vi "Begin.vi"(8 "error in":errorcluster) -> (0 "error out":errorcluster)   [LabVIEW 2016]
doc: "Called before other user functions, this VI is expected to open initial I/O refnums, load in file data, and do all program initialization. Notice that the <B>error out</B> terminal is simply used for data flow. Wiring it to other structures or subVIs ensures that this VI runs first."
uses:
  <vilib>/Rock Robotics/WPI/DriverStation/WPI_DriverStationRobotMode2.ctl
  <vilib>/Rock Robotics/WPI/Joystick/WPI_JoystickDeviceEnum.ctl
  <vilib>/Rock Robotics/SystemInterfaces/DIO/FPGA_DIOPWMChannel.ctl
  <vilib>/Rock Robotics/WPI/SafetyOutput/WPI_SafetyOutputConfigMenu.ctl
  <vilib>/Rock Robotics/WPI/ThirdParty/CanMotor/TalonSRX/WPI_CANTalonSRX_APIControlMode.ctl
  <vilib>/Rock Robotics/WPI/ThirdParty/CanMotor/TalonSRX/WPI_CANTalonSRX_APIFeedbackSelect.ctl
  Robot Global Data.vi
  <vilib>/Rock Robotics/Network Tables/NT Write String Array.vi
  <vilib>/Rock Robotics/Network Tables/NT Write String.vi
  5492_DriveOrientation.vi
  5492_OrientationButtonPress.vi
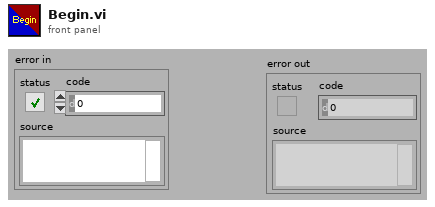
[diagram p1: front panel]
types:
  T1 = typedef "FPGA_DIOPWMChannel.ctl" = enum8{"PWM 0", "PWM 1", "PWM 2", "PWM 3", "PWM 4", "PWM 5", "PWM 6", "PWM 7", "PWM 8", "PWM 9", "PWM MXP 0", "PWM MXP 1", "PWM MXP 2", "PWM MXP 3", "PWM MXP 4", "PWM MXP 5", "PWM MXP 6", "PWM MXP 7", "PWM MXP 8", "PWM MXP 9", "Invalid"}
  T2 = typedef "WPI_CANTalonSRX_APIControlMode.ctl" = enum8{"Percent VBus", "Speed", "Position", "Slave", "Unchanged / Invalid", "Voltage Compensation", "Current", "Motion Profile", "Motion Magic"}
  T3 = typedef "WPI_CANTalonSRX_APIFeedbackSelect.ctl" = enum16{"Digital Quadrature Encoder", "Analog Potentiometer", "Analog Encoder", "Count on Quad-A (Rising-Edge)", "Count on Quad-A (Falling-Edge)", "CTR Magnetic Enc (Absolute)", "CTR Magnetic Enc (Relative)", "Pulse Width"}
  T4 = typedef "WPI_JoystickDeviceEnum.ctl" = enum16{"USB 0", "USB 1", "USB 2", "USB 3", "USB 4", "USB 5"}
  T5 = typedef "WPI_SafetyOutputConfigMenu.ctl" = enum16{"Enable", "Disable"}
  T6 = typedef "WPI_DriverStationRobotMode2.ctl" = enum16{"Autonomous Disabled", "Autonomous Enabled", "Teleop Disabled", "Teleop Enabled", "Disconnected", "Finish", "Test Disabled", "Test Enabled", "Emergency Stopped"}
  T7 = typedef "WPI_JoystickDevRef.ctl" = cluster{"Device":T4}
  T8 = typedef "WPI_MotorControlDeviceRef.ctl" = cluster{"DeviceStatus":errorcluster, "Type":T9, "PWM":cluster{"PWM Channel":T1, "DeadBand":T10}, "CAN":cluster{"Device Number":u8, "SetOutput VI Ref":variant, "GetOutput VI Ref":variant, "Enable VI Ref":variant, "Disable VI Ref":variant, "Data":variant}, "Invert":bool}
  T9 = typedef "WPI_MotorControlType.ctl" = enum16{"PWM", "CAN"}
  T10 = typedef "WPI_PWMDeadband.ctl" = cluster{"Name":string, "maxPositivePwm":i32, "minPositivePwm":i32, "centerPwm":i32, "maxNegativePwm":i32, "minNegativePwm":i32, "angularRange":u16}
  T11 = typedef "WPI_RobotDriveDevRef.ctl" = cluster{"DevStatus":errorcluster, "Motors[]":T8[], "Square Inputs":bool, "Max Output":dbl}
  T12 = typedef "WPI_PWMDeviceRef.ctl" = cluster{"DeviceStatus":errorcluster, "PWM Channel":T1}
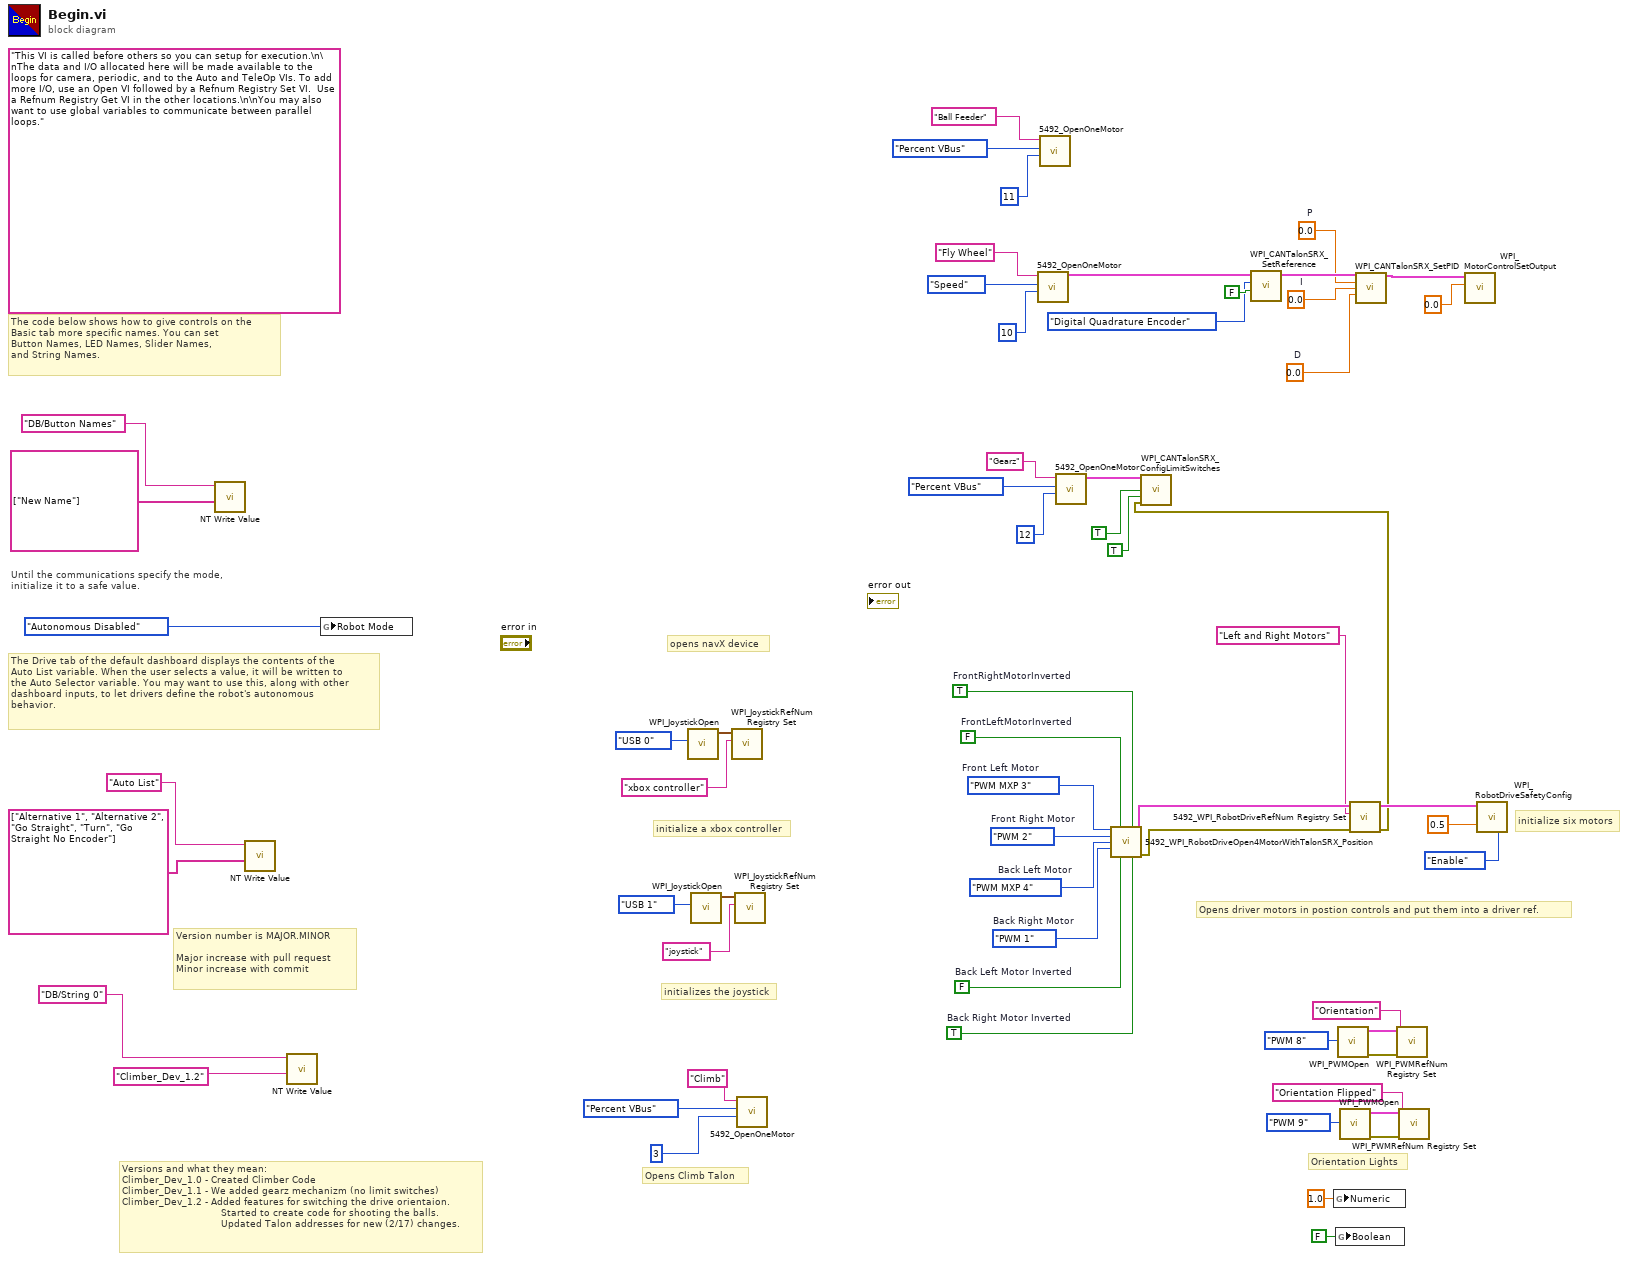
[diagram p0: block diagram]
diagram:
  w16 = 0.0  # D
  w17 = 0.0  # I
  w18 = 0.0  # P
  w43 = TRUE  # Back Right Motor Inverted
  w44 = FALSE  # Back Left Motor Inverted
  w45 = FPGA_DIOPWMChannel."PWM MXP 4"  # Back Left Motor
  w51 = FPGA_DIOPWMChannel."PWM 1"  # Back Right Motor
  w52 = FPGA_DIOPWMChannel."PWM 2"  # Front Right Motor
  w53 = FPGA_DIOPWMChannel."PWM MXP 3"  # Front Left Motor
  w50 = FALSE  # FrontLeftMotorInverted
  w49 = TRUE  # FrontRightMotorInverted
  (unwired) "This VI is called before others so you can setup for execution.\n\nThe data and I/O allocated here will be made available to the loops for camera, periodic, and to the Auto and TeleOp VIs. To add more I/O, use an Open VI followed by a Refnum Registry Set VI.  Use a Refnum Registry Get VI in the other locations.\n\nYou may also want to use global variables to communicate between parallel loops."
  # "Orientation Lights"
  # "Versions and what they mean:\nClimber_Dev_1.0 - Created Climber Code\nClimber_Dev_1.1 - We added gearz mechanizm (no limit switches)\nClimber_Dev_1.2 - Added features for switching the drive orientaion.\n                                 Started to create code for shooting the balls.\n                                 Updated Talon addresses for new (2/17) changes."
  # "Opens Climb Talon"
  # "Version number is MAJOR.MINOR\n\nMajor increase with pull request\nMinor increase with commit"
  # "opens navX device"
  # "Opens driver motors in postion controls and put them into a driver ref."
  # "initializes the joystick"
  # "initialize six motors"
  # "The Drive tab of the default dashboard displays the contents of the\nAuto List variable. When the user selects a value, it will be written to\nthe Auto Selector variable. You may want to use this, along with other\ndashboard inputs, to let drivers define the robot's autonomous\nbehavior."
  # "The code below shows how to give controls on the\nBasic tab more specific names. You can set\nButton Names, LED Names, Slider Names,\nand String Names."
  # "initialize a xbox controller"
  # "Until the communications specify the mode,\ninitialize it to a safe value."
  n1 = call-poly <vilib>:"NT Write Value.vi"("String Array"=string[] ["New Name"], "Name"="DB/Button Names") -> ()  [unwired: 9 in, 1 out]
  n2 = call-poly <vilib>:"NT Write Value.vi"("String Array"=string[] ["Alternative 1", "Alternative 2", "Go Straight", "Turn", "Go Straight No Encoder"], "Name"="Auto List") -> ()  [unwired: 9 in, 1 out]
  n3 = call-poly <vilib>:"NT Write Value.vi"("String"="Climber_Dev_1.2", "Name"="DB/String 0") -> ()  [unwired: 9 in, 1 out]
  n4 = global write "Robot Global Data.vi" "Robot Mode"(WPI_DriverStationRobotMode2."Autonomous Disabled" ("Robot Mode")) -> ()
  n5 = call <vilib>:"WPI_JoystickOpen.vi"("JoystickDevice"=WPI_JoystickDeviceEnum."USB 0") -> ("JoystickDevRef"=w60:T7)  [unwired: 10 in]
  n6 = call <vilib>:"WPI_JoystickOpen.vi"("JoystickDevice"=WPI_JoystickDeviceEnum."USB 1") -> ("JoystickDevRef"=w40:T7)  [unwired: 10 in]
  n7 = call <vilib>:"WPI_JoystickRefNum Registry Set.vi"("refnum name"="xbox controller", "JoystickDevRef"=w60) -> ()  [unwired: 8 in, 2 out]
  n8 = call <vilib>:"WPI_JoystickRefNum Registry Set.vi"("refnum name"="joystick", "JoystickDevRef"=w40) -> ()  [unwired: 8 in, 2 out]
  n9 = call "5492_OpenOneMotor.vi"("Device Number"=u8 3, "Control Mode"=WPI_CANTalonSRX_APIControlMode."Percent VBus", "refnum name"="Climb") -> ()  [unwired: 7 in, 2 out]
  n10 = call "5492_OpenOneMotor.vi"("Device Number"=u8 10, "Control Mode"=WPI_CANTalonSRX_APIControlMode."Speed", "refnum name"="Fly Wheel") -> ("MotorControlDevRef"=w20:T8)  [unwired: 7 in, 1 out]
  n11 = call "5492_OpenOneMotor.vi"("Device Number"=u8 11, "Control Mode"=WPI_CANTalonSRX_APIControlMode."Percent VBus", "refnum name"="Ball Feeder") -> ()  [unwired: 7 in, 2 out]
  n12 = call "5492_OpenOneMotor.vi"("Device Number"=u8 12, "Control Mode"=WPI_CANTalonSRX_APIControlMode."Percent VBus", "refnum name"="Gearz") -> ("MotorControlDevRef"=w29:T8)  [unwired: 7 in, 1 out]
  n13 = call "5492_WPI_RobotDriveOpen4MotorWithTalonSRX_Position.vi"("Front Left Motor"=w53, "Front Left Motor Inverted"=w50, "Front Right Motor Inverted"=w49, "Front Right Motor"=w52, "Back Left Motor"=w45, "Back Right Motor"=w51, "Back Left Motor Inverted"=w44, "Back Right Motor Inverted"=w43) -> ("RobotDriveDevRef"=w48:T11, "error out"=w47:errorcluster)  [unwired: 6 in]
  n14 = call <vilib>:"WPI_CANTalonSRX_SetReference.vi"("Reverse Feedback Sensor"=FALSE, "Feedback Reference"=WPI_CANTalonSRX_APIFeedbackSelect."Digital Quadrature Encoder", "CAN Talon SRX Ref"=w20) -> ("CAN Talon SRX Ref"=w19:T8)  [unwired: 7 in, 1 out]
  n15 = global write "5492_DriveOrientation.vi" "Numeric"(1.0 ("Numeric")) -> ()
  n16 = global write "5492_OrientationButtonPress.vi" "Boolean"(FALSE ("Boolean")) -> ()
  n17 = call <vilib>:"WPI_PWMOpen.vi"("PWM Channel"=FPGA_DIOPWMChannel."PWM 8") -> ("error out"=w8:errorcluster, "PWMDeviceRef"=w7:T12)  [unwired: 9 in]
  n18 = call <vilib>:"WPI_PWMOpen.vi"("PWM Channel"=FPGA_DIOPWMChannel."PWM 9") -> ("error out"=w1:errorcluster, "PWMDeviceRef"=w2:T12)  [unwired: 9 in]
  n19 = call "5492_WPI_RobotDriveRefNum Registry Set.vi"("error in (no error)"=w47, "refnum name"="Left and Right Motors", "RobotDriveDevRef"=w48) -> ("error out"=w26:errorcluster, "RobotDriveDevRef"=w42:T11)  [unwired: 1 in, 6 out]
  n20 = call <vilib>:"WPI_CANTalonSRX_ConfigLimitSwitches.vi"("CAN Talon SRX Ref"=w29, "Forward Limit Switch Normally Open"=TRUE, "Reverse Limit Switch Normally Open"=TRUE, "error in (no error)"=w26) -> ()  [unwired: 10 in, 2 out]
  n21 = call <vilib>:"WPI_CANTalonSRX_SetPID.vi"("CAN Talon SRX Ref"=w19, "P"=w18, "I"=w17, "D"=w16) -> ("CAN Talon SRX Ref"=w15:T8)  [unwired: 10 in, 1 out]
  n22 = call <vilib>:"WPI_PWMRefNum Registry Set.vi"("error in (no error)"=w8, "refnum name"="Orientation", "PWMDeviceRef"=w7) -> ()  [unwired: 7 in, 2 out]
  n23 = call <vilib>:"WPI_PWMRefNum Registry Set.vi"("error in (no error)"=w1, "refnum name"="Orientation Flipped", "PWMDeviceRef"=w2) -> ()  [unwired: 7 in, 2 out]
  n24 = call <vilib>:"WPI_MotorControlSetOutput.vi"("Output"=0.0, "MotorControlDevRef"=w15) -> ()  [unwired: 7 in, 3 out]
  n25 = call <vilib>:"WPI_RobotDriveSafetyConfig.vi"("timeout (s)"=0.5, "mode"=WPI_SafetyOutputConfigMenu."Enable", "RobotDriveDevRef"=w42) -> ()  [unwired: 7 in, 2 out]
